vi "Refrsh2DGraphArrDev.vi"(8 "error in (no error)":errorcluster caption="entrée d'erreur (pas d'erreur)", 9 "CurveIndex":i32, 10 "PointIndex":i32, 11 "Interface en entrée":refnum<class "Interface.lvclass"> caption="DNL_LabVIEW Object in") -> (0 "error out":errorcluster caption="sortie d'erreur", 3 "Interface en sortie":refnum<class "Interface.lvclass"> caption="DNL_LabVIEW Object out")   [LabVIEW 2019, in "Interface.lvclass"]
uses:
  Interface.lvclass
  2DGraphQData.ctl
  Experiment Class/ArrDevData.ctl
panel:
  in  "2DGphInd":i32
  in  "ArrDevDat":T1={"MeasDatOut"=array1024x3[3072 elements], "XDatOut"=array1024x2[2048 elements], "YDatOut"=[[1.0], [2.0], [3.0]], "DevID"=1}
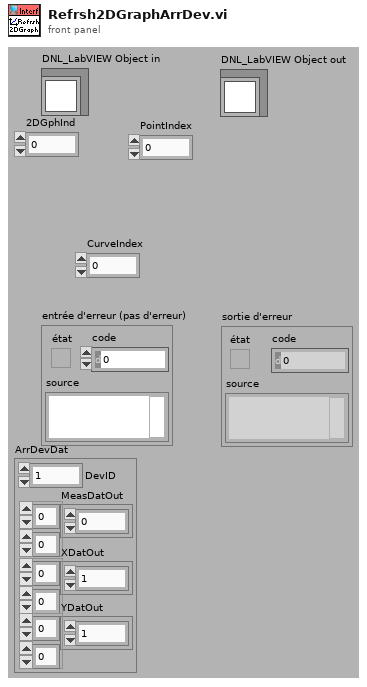
[diagram p1: front panel]
types:
  T1 = typedef "ArrDevData.ctl" = cluster{"MeasDatOut":dbl[][], "XDatOut":dbl[][], "YDatOut":dbl[][], "DevID":i32}
  T2 = typedef "2DGraphQData.ctl" = cluster{"X Ind(Line)":i32, "Y Ind(Col)":i32, "Data":dbl}
  T3 = typedef "2DGraphSetup.ctl" = cluster{"ZDataIndex":i32, "XParIndex":i32, "YParIndex":i32, "FillLineFirst":bool, "2DGraphIndex":i32, "XParQ Ref":refnum<queue>, "YParQ Ref":refnum<queue>, "DataQRefs":refnum<queue>[]}
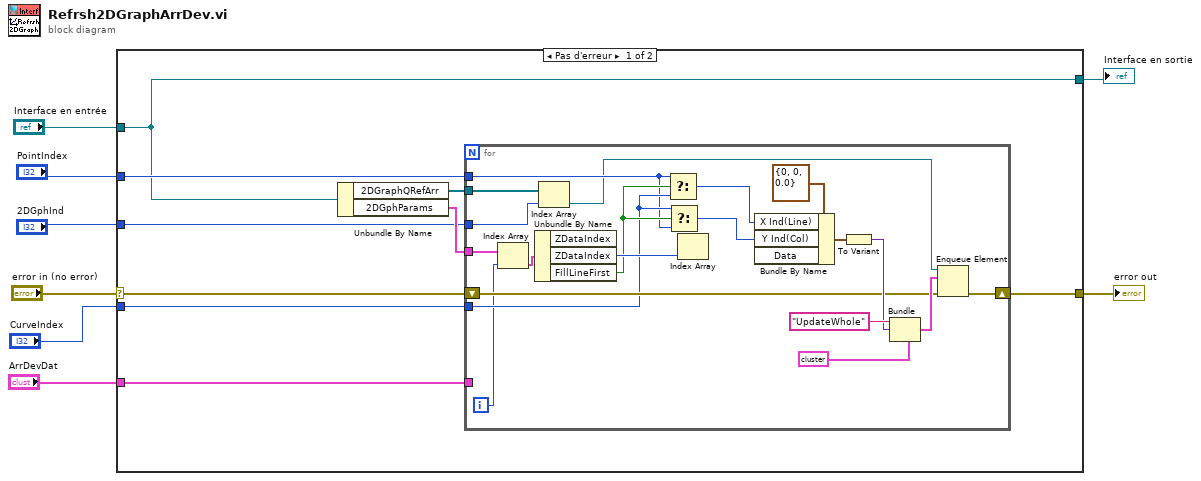
[diagram p0: block diagram]
diagram:
  n1 = case shown="Pas d'erreur" "error in (no error)" {
    selector: "error in (no error)" -> [w17 w39]
    tunnel: [w16 w39] -> w7
    tunnel: [w12 w38] -> w5
    tunnel: "Interface en entrée" -> [w12 w38]
    tunnel: "CurveIndex" -> [w15 _]
    tunnel: "ArrDevDat" -> [w14 _]
    tunnel: "PointIndex" -> [w13 _]
    tunnel: "2DGphInd" -> [w9 _]
    frame No Error {
      n2 = Unbundle By Name(w12) -> ("2DGraphQRefArr"=w11:refnum<queue>[], "2DGphParams"=w10:T3[])
      n3 = for {
        tunnel: w9 -> [w31]
        shift-right: [w32] -> w16
        shift-left: w17 -> [w23]
        tunnel: w10 -> [w37]
        tunnel: w15 -> [w22]
        tunnel: w11 -> [w30]
        tunnel: w14 -> [_]
        tunnel: w13 -> [w21]
        i -> [w18]
        n4 = Index Array(array=w37, index=w18) -> (element=w36:T3)
        n5 = Unbundle By Name(w36) -> ("ZDataIndex"=w29:i32, "FillLineFirst"=w25:bool)  [unwired: 1 out]
        n6 = Index Array(array=w30, index=w31) -> (element=w19:refnum<queue>)
        n7 = Select(t=w21, s=w25, f=w22) -> (s? t:f=w24:i32)
        n8 = Select(t=w22, s=w25, f=w21) -> (s? t:f=w20:i32)
        n9 = Index Array(index=w29) -> ()  [unwired: 1 in, 1 out]
        n10 = Bundle By Name(cluster=T2 {"X Ind(Line)"=0, "Y Ind(Col)"=0, "Data"=0.0} ("2DGphQData"), "X Ind(Line)"=w24, "Y Ind(Col)"=w20) -> (w27:T2)  [unwired: 1 in]
        n11 = To Variant(anything=w27) -> (Variant=w26:variant)
        n12 = Bundle(cluster=cluster{"Message":string, "Data":variant, i32} {"Message"="", "Data"=variant, 0} ("élément"), "Message"="UpdateWhole", "Data"=w26) -> (w34:cluster{"Message":string, "Data":variant, i32})  [unwired: 1 in]
        n13 = Enqueue Element(queue=w19, element=w34, error in (no error)=w23) -> (error out=w32:errorcluster)  [unwired: 1 in, 2 out]
      }
    }
    frame Error {
    }
  }
  "error out" <- w7
  "Interface en sortie" <- w5
